vi "eFGV - DI Data RT.vi"(6 "States":T1, 8 "Error In":errorcluster, 11 "DI Data In":digitalwaveform[](array[waveform])) -> (0 "Error Out":errorcluster, 3 "DI Data Out":refnum<user-event>)   [LabVIEW 2020]
uses:
  Control/State - eFGV.ctl
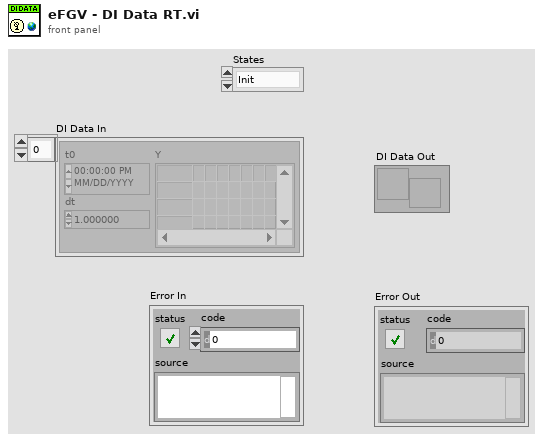
[diagram p1: front panel]
types:
  T1 = typedef "State - eFGV.ctl" = enum16{"Init", "Read", "Write", "Exit"}
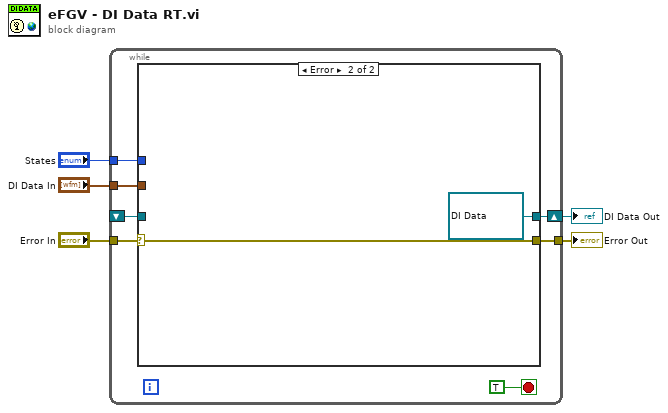
[diagram p0: block diagram]
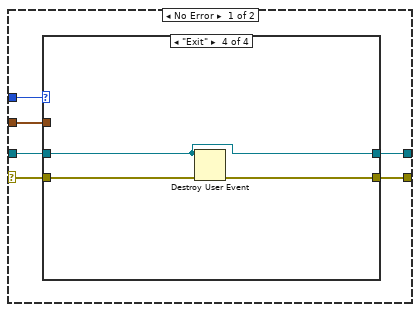
[diagram p2: hidden frame]
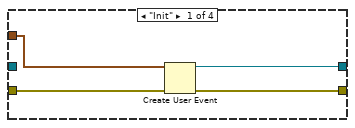
[diagram p3: hidden frame]
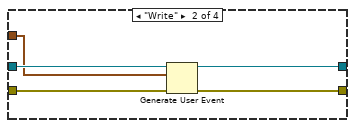
[diagram p4: hidden frame]
diagram:
  n1 = while {
    tunnel: "Error In" -> [w11]
    tunnel: [w10] -> w4
    tunnel: "States" -> [w9]
    tunnel: "DI Data In" -> [w8]
    shift-right: [w7] -> w1
    shift-left: _ -> [w6]
    stop <- TRUE stop-if-true
    n2 = case shown="Error" w11 {
      selector: w11 -> [w17 w34]
      tunnel: [w16 w34] -> w10
      tunnel: w9 -> [w18 _]
      tunnel: w8 -> [w15 _]
      tunnel: [w14 refnum<user-event> refnum ("DI Data In")] -> w7
      tunnel: w6 -> [w13 _]
      frame No Error {
        n3 = case shown="\"Exit\"" w18 {
          tunnel: w17 -> [w22 w27 w29 w32]
          tunnel: [w21 w26 w29 w31] -> w16
          tunnel: w15 -> [w20 w23 _ _]
          tunnel: [w19 w24 w28 w30] -> w14
          tunnel: w13 -> [_ w25 w28 w30]
          frame "Init" {
            n4 = Create User Event(user event datatype=w20, error in=w22) -> (user event=w19:refnum<user-event>, error out=w21:errorcluster)
          }
          frame "Write" {
            n5 = Generate User Event(user event=w25, event data cluster=w23, error in=w27) -> (user event out=w24:refnum<user-event>, error out=w26:errorcluster)  [unwired: 1 in]
          }
          frame "Read" {
          }
          frame "Exit" {
            n6 = Destroy User Event(user event=w30, error in=w32) -> (error out=w31:errorcluster)
          }
        }
      }
      frame Error {
      }
    }
  }
  "Error Out" <- w4
  "DI Data Out" <- w1
